vi "Write Graph.vi"(8 "error in (no error)":errorcluster, 10 "Graph":T1, 11 "I-V Result in":refnum<class "I-V Result.lvclass">) -> (0 "error out":errorcluster, 3 "I-V Result out":refnum<class "I-V Result.lvclass">)   [LabVIEW 2013, in "Diode Characterization.lvlib" / "I-V Result.lvclass"]
uses:
  I-V Result.lvclass
  graphdata.ctl
  <vilib>/Utility/miscctls.llb/LVAnnotationListTypeDef.ctl
  <vilib>/Utility/miscctls.llb/LVCursorListTypeDef.ctl
  I-V Result.lvclass/I-V Result.ctl
  Diode IV.lvclass
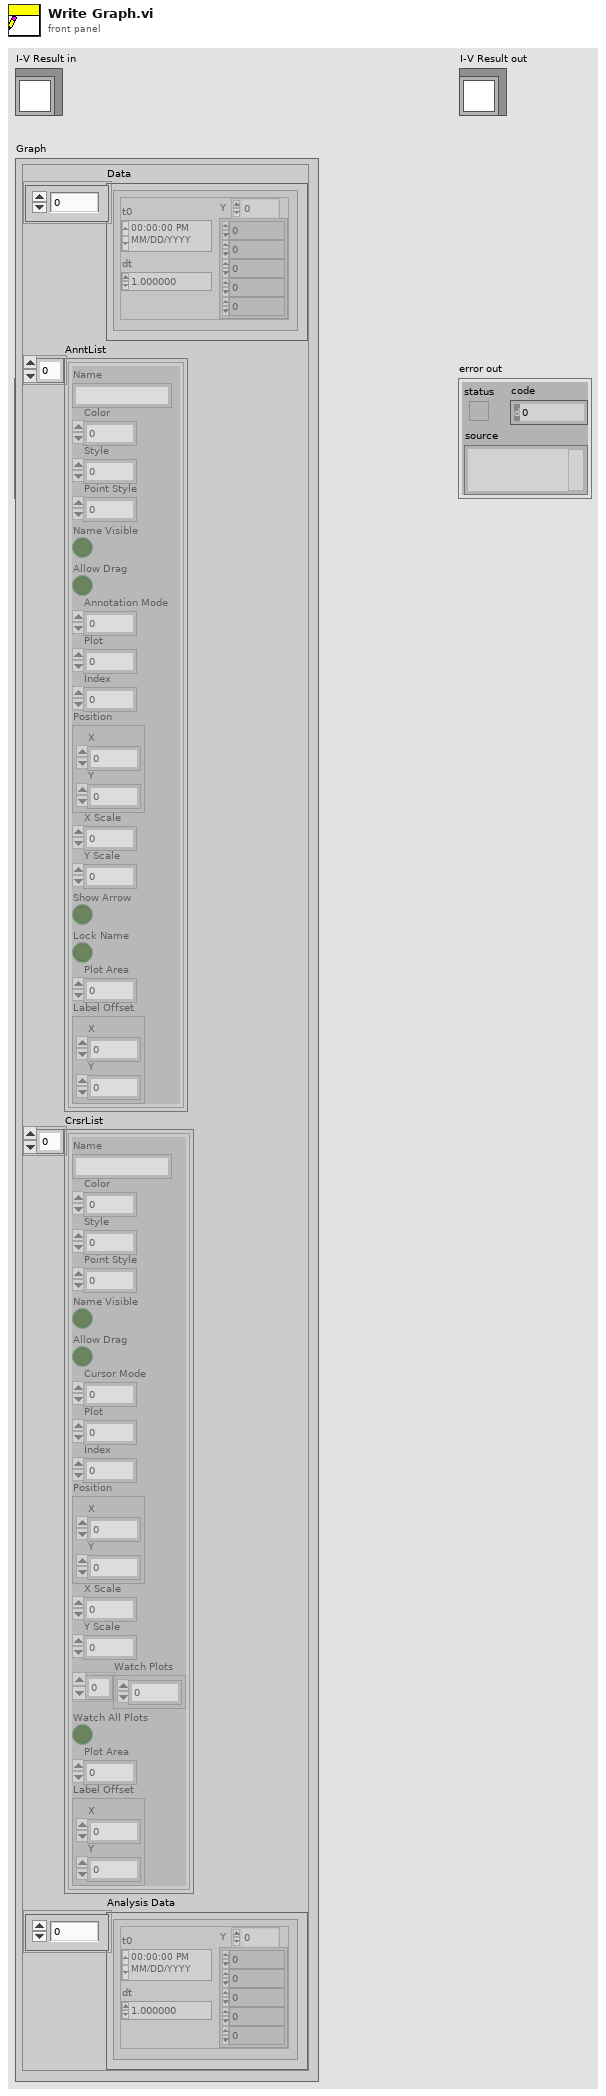
[diagram p1: front panel]
types:
  T1 = typedef "Diode Characterization.lvlib/Diode IV.lvclass/graphdata.ctl" = cluster{"Data":waveform(dbl)[], "AnntList":T2, "CrsrList":T3, "Analysis Data":waveform(dbl)[]}
  T2 = typedef "LVAnnotationListTypeDef.ctl" = cluster{"Name":string, "Color":u32, "Style":u8, "Point Style":u8, "Name Visible":bool, "Allow Drag":bool, "Annotation Mode":u32, "Plot":i32, "Index":i32, "Position":cluster{"X":dbl, "Y":dbl}, "X Scale":u32, "Y Scale":u32, "Show Arrow":bool, "Lock Name":bool, "Plot Area":i32, "Label Offset":cluster{"X":dbl, "Y":dbl}}[]
  T3 = typedef "LVCursorListTypeDef.ctl" = cluster{"Name":string, "Color":u32, "Style":u8, "Point Style":u8, "Name Visible":bool, "Allow Drag":bool, "Cursor Mode":u32, "Plot":i32, "Index":i32, "Position":cluster{"X":dbl, "Y":dbl}, "X Scale":u32, "Y Scale":u32, "Watch Plots":i32[], "Watch All Plots":bool, "Plot Area":i32, "Label Offset":cluster{"X":dbl, "Y":dbl}}[]
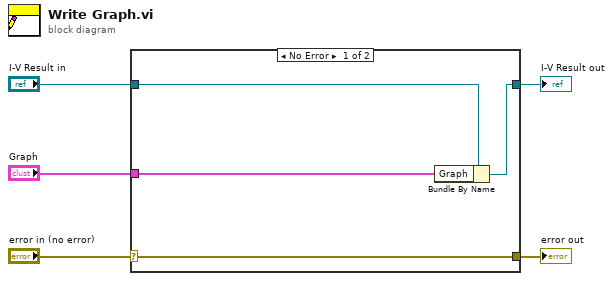
[diagram p0: block diagram]
diagram:
  n1 = case shown="No Error" "error in (no error)" {
    selector: "error in (no error)" -> [w9 w10]
    tunnel: [w9 w10] -> w4
    tunnel: [w7 w11] -> w2
    tunnel: "I-V Result in" -> [w8 w11]
    tunnel: "Graph" -> [w6 _]
    frame No Error {
      n2 = Bundle By Name(cluster=w8, "Graph"=w6) -> (w7:refnum<class "I-V Result.lvclass">)
    }
    frame Error {
    }
  }
  "error out" <- w4
  "I-V Result out" <- w2
